vi "Enqueue.vi"(8 "error in (no error)":errorcluster, 10 "Message in":refnum<class "Abstract Message.lvclass">, 11 "Message Queue in":refnum<class "Message Queue.lvclass">) -> (0 "error out":errorcluster, 3 "Message Queue out":refnum<class "Message Queue.lvclass">)   [LabVIEW 2017, in "Messaging.lvlib" / "Message Queue.lvclass"]
uses:
  Message Queue.lvclass
  Message/Abstract Message/Abstract Message.lvclass
  Message Queue.lvclass/Message Queue.ctl
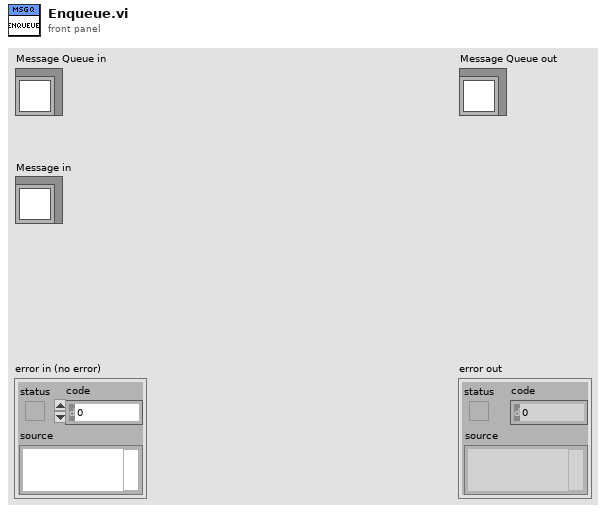
[diagram p1: front panel]
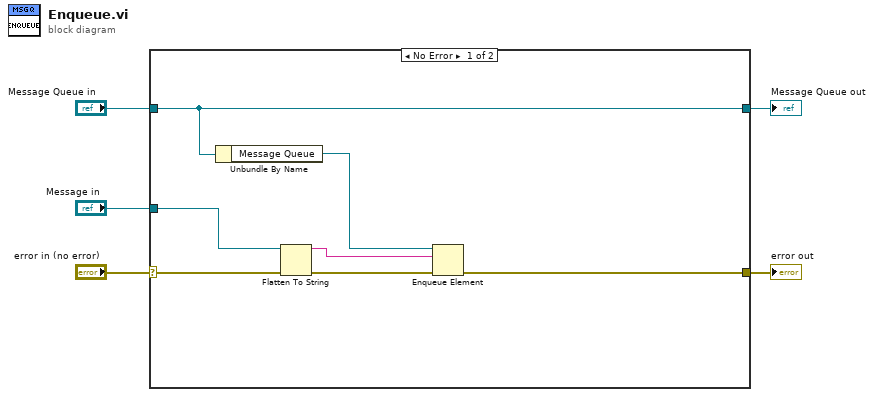
[diagram p0: block diagram]
diagram:
  n1 = case shown="No Error" "error in (no error)" {
    selector: "error in (no error)" -> [w7 w14]
    tunnel: [w12 w14] -> w4
    tunnel: [w11 w13] -> w2
    tunnel: "Message Queue in" -> [w11 w13]
    tunnel: "Message in" -> [w9 _]
    frame No Error {
      n2 = Unbundle By Name(w11) -> ("Message Queue"=w10:refnum<queue>)
      n3 = Flatten To String(anything=w9, error in (no error)=w7) -> (data string=w8:string, error out=w6:errorcluster)  [unwired: 2 in, 1 out]
      n4 = Enqueue Element(queue=w10, element=w8, error in (no error)=w6) -> (error out=w12:errorcluster)  [unwired: 1 in, 2 out]
    }
    frame Error {
    }
  }
  "error out" <- w4
  "Message Queue out" <- w2
